vi "Scheduler.Service.vi"(11 "Parent Q":refnum<queue>) -> ()   [LabVIEW 2024, in "EQMF.lvlib" / "Scheduler.lvlib"]
uses:
  Scheduler.lvlib
  Queues/Q.Element.ctl
  Queues/Queue Utils.lvlib
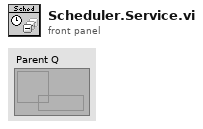
[diagram p1: front panel]
types:
  T1 = typedef "EQMF.lvlib/Queue Utils.lvlib/Q.Element.ctl" = cluster{"Cmd":string, "Sub":string, "Data1":variant, "Data2":variant}
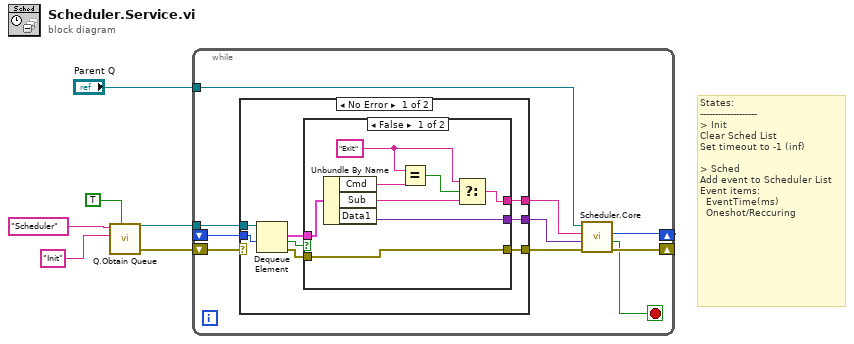
[diagram p0: block diagram]
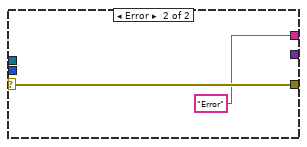
[diagram p3: hidden frame]
diagram:
  # "States:\n-------------------\n> Init\nClear Sched List\nSet timeout to -1 (inf)\n\n> Sched\nAdd event to Scheduler List\nEvent items:\n  EventTime(ms)\n  Oneshot/Reccuring"
  n1 = call "Q.Obtain Queue.vi"("Enqueue Init"=TRUE, "Init.Sub"="Init" ("name (unnamed)"), "Q Name"="Scheduler" ("name (unnamed)")) -> ("error out"=w5:errorcluster, "Q Out"=w6:refnum<queue>)  [unwired: 6 in, 1 out]
  n2 = while {
    tunnel: w6 -> [w16]
    tunnel: "Parent Q" -> [w12]
    shift-right: [w8] -> _
    shift-left: w5 -> [w15]
    shift-right: [w9] -> _
    shift-left: _ -> [w14]
    stop <- w7 stop-if-true
    n3 = case shown="No Error" w15 {
      selector: w15 -> [_ w35]
      tunnel: w16 -> [w24 _]
      tunnel: [w20 "Error"] -> w13
      tunnel: [w21 _] -> w10
      tunnel: [w17 w35] -> w11
      tunnel: w14 -> [w23 _]
      frame No Error {
        n4 = Dequeue Element(queue=w24, timeout in ms (-1)=w23) -> (element=w22:T1, timed out?=w19:bool, error out=w18:errorcluster)  [unwired: 1 in, 1 out]
        n5 = case shown="False" w19 {
          tunnel: w22 -> [w32 _]
          tunnel: [w31 _] -> w21
          tunnel: [w25 _] -> w20
          tunnel: w18 -> [w30 w33]
          tunnel: [w30 w33] -> w17
          frame False {
            w27 = "Exit" ("x")
            n6 = Unbundle By Name(w32) -> ("Cmd"=w29:string, "Sub"=w26:string, "Data1"=w31:variant)
            n7 = Equal?(x=w27, y=w29) -> (x = y?=w28:bool)
            n8 = Select(t=w27, s=w28, f=w26) -> (s? t:f=w25:string)
          }
          frame True {
          }
        }
      }
      frame Error {
      }
    }
    n9 = call "Scheduler.Core.vi"("Error In"=w11, "Data"=w10, "Cmd"=w13, "Parent Q"=w12) -> ("Error Out"=w8:errorcluster, "Exit"=w7:bool, "Remaining ms"=w9:i32)  [unwired: 4 in, 1 out]
  }
